vi "Progress.vi"() -> ()   [LabVIEW 2010]
panel:
  out "Progress multiple %":u8(slide) max=100 step=1 scale=0.0..100.0
  out "Stop":bool
  out "Progress%":u8(slide) max=100 step=1 scale=0.0..100.0
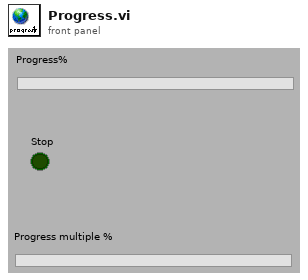
[diagram p1: front panel]
diagram:
